vi "GetChartParams.vi"(8 "error in (no error)":errorcluster, 10 "GraphInfoCluster":T1={"RT Display Reader Loop Time [us]"=1000, "Sensor Gains [um/V]"={"G_SE"=1.0, "G_NE"=1.0, "G_NW"=1.0, "G_SW"=1.0, "G_CI"=1.0}, "Sensor H-Offset  [mm]"={"X"=1.0, "Y"=1.0}, "Amplifier Gains [V/V]"={"G_SE"=1.0, "G_NE"=1.0, "G_NW"=1.0, "G_SW"=1.0, "G_CO"=1.0, "G_CI"=1.0}, "Curr Sense Gain [mA/V]"={"G_CS"=0.0}}, 11 "DisplayWaveforms":refnum<class "DisplayWaveforms.lvclass">) -> (0 "error out":errorcluster, 2 "ChartParams":T7={"Chart ScaleMultipliers"={"WF Xscale Multiplier"=0.0, "WF Yscale Multiplier"=[]}, "Coord Transform Multipliers"={"Z-Multiplier"=1.0, "Th-Multiplier"=0.0}}, 3 "DisplayWaveforms out":refnum<class "DisplayWaveforms.lvclass">)   [LabVIEW 2020, in "DisplayWaveform.lvlib" / "DisplayWaveforms.lvclass"]
doc: "Get Chart Attributes to send to Chart UI"
uses:
  DisplayWaveforms.lvclass
  Controller/TypeDefs/ChartParamsCluster.ctl
  Controller/TypeDefs/GraphInfoCluster.ctl
  Controller/TypeDefs/RTdisplayTimedLoop_dt.ctl
  Controller/TypeDefs/SensorGains.ctl
  Controller/TypeDefs/SensorHposOffset.ctl
  Controller/TypeDefs/AmplifierGains.ctl
  Controller/TypeDefs/CurrSenseGains.ctl
  <vilib>/Analysis/baseanly.llb/Mean (DBL).vi
  DisplayWaveforms.lvclass/DisplayWaveforms.ctl
  <vilib>/Analysis/NI_AALBase.lvlib
panel:
  # "For instructions on how to use the JKI State Machine Objects, examples and video tutorials, visit:\nhttp://jki.net/state-machine-objects/\n\nJKI State Machine Objects™\nhttp://jki.net/state-machine-objects/\nCopyright (C) 2005-2015, JKI <info@jki.net>\nALL RIGHTS RESERVED"
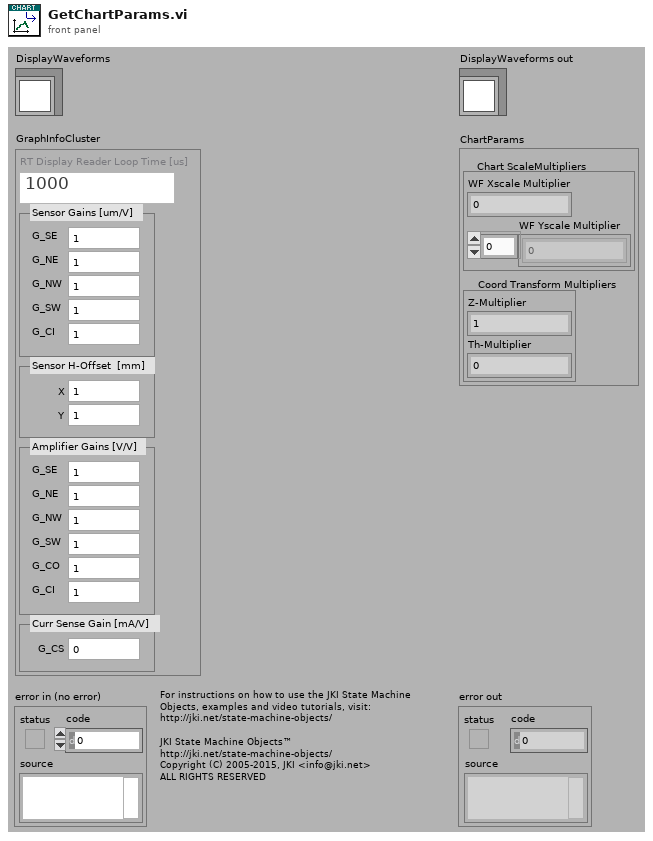
[diagram p1: front panel]
types:
  T1 = typedef "GraphInfoCluster.ctl" = cluster{"RT Display Reader Loop Time [us]":T2, "Sensor Gains [um/V]":T3, "Sensor H-Offset  [mm]":T4, "Amplifier Gains [V/V]":T5, "Curr Sense Gain [mA/V]":T6}
  T2 = typedef "RTdisplayTimedLoop_dt.ctl" = i64
  T3 = typedef "SensorGains.ctl" = cluster{"G_SE":dbl, "G_NE":dbl, "G_NW":dbl, "G_SW":dbl, "G_CI":dbl}
  T4 = typedef "SensorHposOffset.ctl" = cluster{"X":dbl, "Y":dbl}
  T5 = typedef "AmplifierGains.ctl" = cluster{"G_SE":dbl, "G_NE":dbl, "G_NW":dbl, "G_SW":dbl, "G_CO":dbl, "G_CI":dbl}
  T6 = typedef "CurrSenseGains.ctl" = cluster{"G_CS":dbl}
  T7 = typedef "ChartParamsCluster.ctl" = cluster{"Chart ScaleMultipliers":cluster{"WF Xscale Multiplier":dbl, "WF Yscale Multiplier":dbl[]}, "Coord Transform Multipliers":cluster{"Z-Multiplier":dbl, "Th-Multiplier":dbl}}
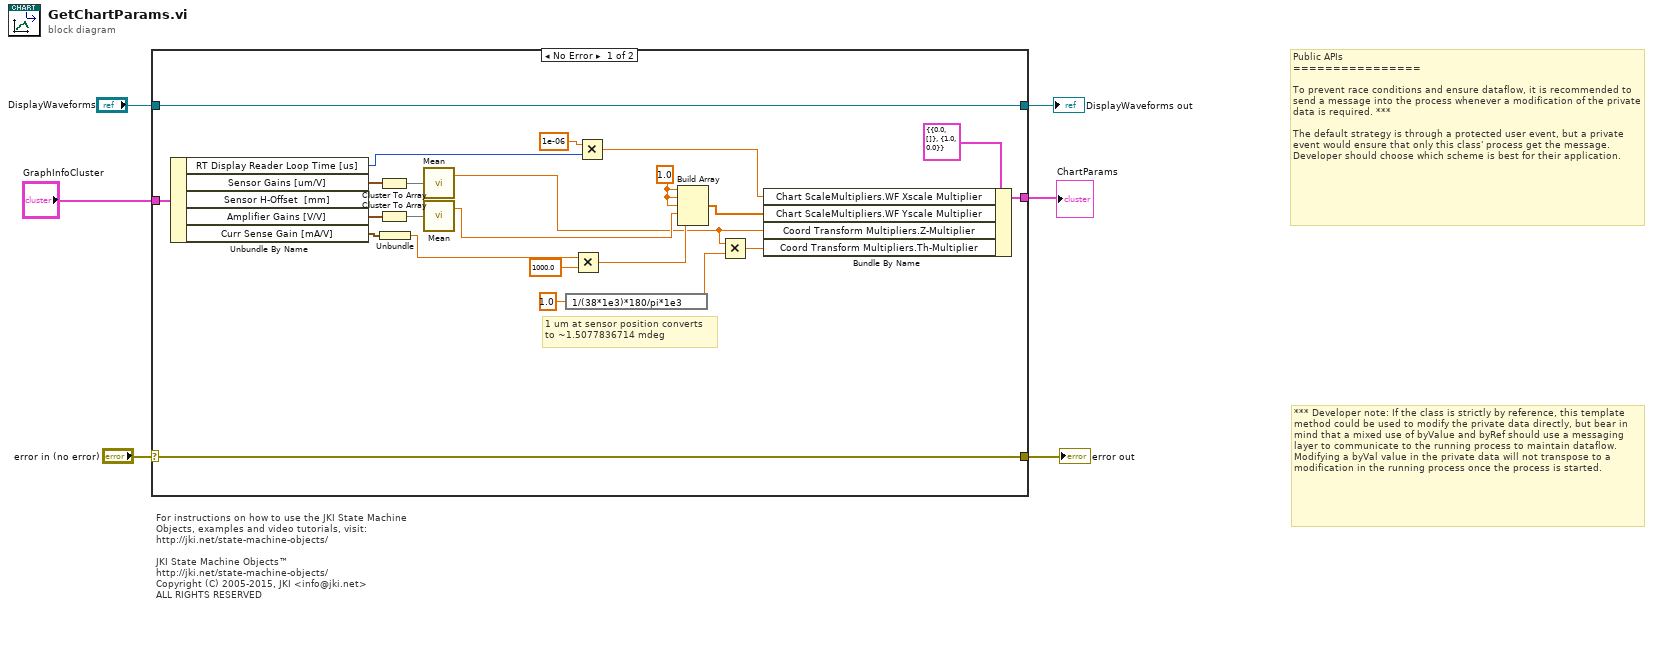
[diagram p0: block diagram]
diagram:
  # "*** Developer note: If the class is strictly by reference, this template method could be used to modify the private data directly, but bear in mind that a mixed use of byValue and byRef should use a messaging layer to communicate to the running process to maintain dataflow. Modifying a byVal value in the private data will not transpose to a modification in the running process once the process is started."
  # "Public APIs\n================\n\nTo prevent race conditions and ensure dataflow, it is recommended to send a message into the process whenever a modification of the private data is required. ***\n\nThe default strategy is through a protected user event, but a private event would ensure that only this class' process get the message. Developer should choose which scheme is best for their application."
  # "For instructions on how to use the JKI State Machine Objects, examples and video tutorials, visit:\nhttp://jki.net/state-machine-objects/\n\nJKI State Machine Objects™\nhttp://jki.net/state-machine-objects/\nCopyright (C) 2005-2015, JKI <info@jki.net>\nALL RIGHTS RESERVED"
  n1 = case shown="No Error" "error in (no error)" {
    selector: "error in (no error)" -> [w14 w30]
    tunnel: "DisplayWaveforms" -> [w29 w31]
    tunnel: [w14 w30] -> w5
    tunnel: [w29 w31] -> w4
    tunnel: "GraphInfoCluster" -> [w28 _]
    tunnel: [w27 _] -> w1
    frame No Error {
      w11 = 1.0 ("element")
      # "1 um at sensor position converts\nto ~1.5077836714 mdeg"
      n2 = Unbundle By Name(w28) -> ("RT Display Reader Loop Time [us]"=w24:T2, "Sensor Gains [um/V]"=w12:T3, "Amplifier Gains [V/V]"=w21:T5, "Curr Sense Gain [mA/V]"=w17:T6)  [unwired: 1 out]
      n3 = Cluster To Array(cluster=w12) -> (array=w13:dbl[])
      n4 = Cluster To Array(cluster=w21) -> (array=w20:dbl[])
      n5 = Unbundle(w17) -> ("G_CS"=w16:dbl)
      n6 = call-poly <vilib>:"Mean.vi"("X"=w13) -> ("mean"=w9:dbl)  [unwired: 1 out]
      n7 = call-poly <vilib>:"Mean.vi"("X"=w20) -> ("mean"=w19:dbl)  [unwired: 1 out]
      n8 = expression code="1/(38*1e3)*180/pi*1e3"(1.0) -> (w7:dbl)
      n9 = Multiply(x=w16, y=1000.0) -> (x*y=w18:dbl)
      n10 = Multiply(x=1e-06, y=w24) -> (x*y=w25:dbl)
      n11 = Build Array(w11, w11, w11, w19, w18) -> (w22:dbl[])
      n12 = Multiply(x=w9, y=w7) -> (x*y=w10:dbl)
      n13 = Bundle By Name(cluster=T7 {"Chart ScaleMultipliers"={"WF Xscale Multiplier"=0.0, "WF Yscale Multiplier"=[]}, "Coord Transform Multipliers"={"Z-Multiplier"=1.0, "Th-Multiplier"=0.0}} ("ChartParams"), "Chart ScaleMultipliers.WF Xscale Multiplier"=w25, "Chart ScaleMultipliers.WF Yscale Multiplier"=w22, "Coord Transform Multipliers.Z-Multiplier"=w9, "Coord Transform Multipliers.Th-Multiplier"=w10) -> (w27:T7)
    }
    frame Error {
    }
  }
  "error out" <- w5
  "DisplayWaveforms out" <- w4
  "ChartParams" <- w1
